vi "Joint Saturation Demo.vi"(10 "Joint Bounds [Deg/mm]":dbl[][](array[numeric])=[[-10.0, 35.0, 0.0, 0.0], [-35.0, -35.0, 0.0, 0.0], [0.5, 10.0, 0.0, 0.0], [-40.0, 40.0, 0.0, 0.0]], 11 "Ref Array [Deg/mm]":dbl[](array[numeric])=[0.0, 0.0, 0.0, 0.0]) -> (2 "Out of Bound?":bool, 3 "Sat Ref Array [Deg/mm]":dbl[](array[numeric]))   [LabVIEW 2016]
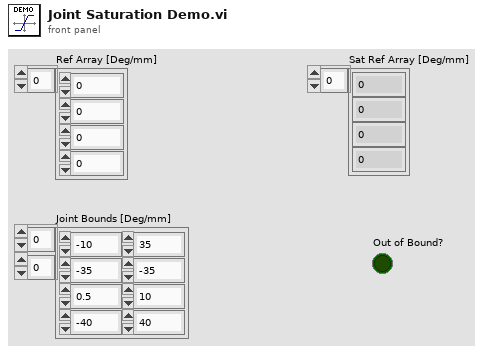
[diagram p1: front panel]
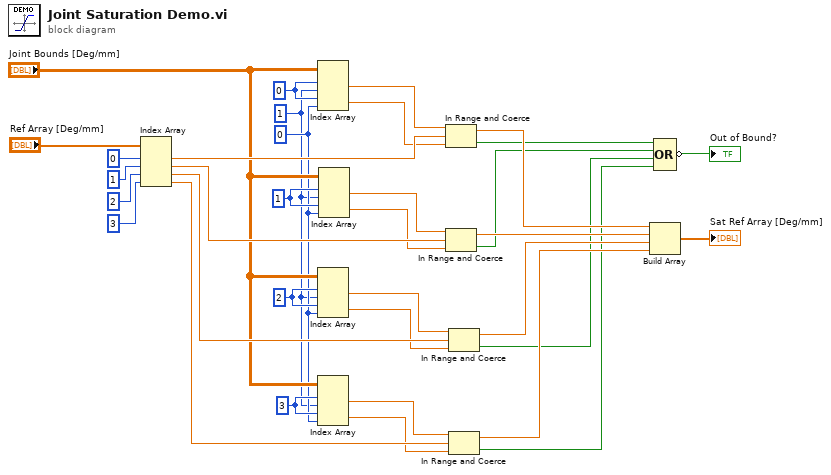
[diagram p0: block diagram]
diagram:
  w10 = 3 ("index (row)")
  w14 = 2
  w21 = 1 ("index (row)")
  w8 = 1 ("disabled index (col)")
  w9 = 0 ("index")
  w25 = 0 ("index")
  n1 = Index Array(array="Ref Array [Deg/mm]", index #1=0 ("index"), index #2=1 ("index"), index #3=2 ("index"), index #4=3 ("index")) -> (element #1=w29:dbl, element #2=w28:dbl, element #3=w27:dbl, element #4=w26:dbl)
  n2 = Index Array(array="Joint Bounds [Deg/mm]", index (row) #1=w25, index (col) #1=w8, index (row) #2=w25, index (col) #2=w9) -> (element #1=w24:dbl, element #2=w23:dbl)
  n3 = Index Array(array="Joint Bounds [Deg/mm]", index (row) #1=w14, index (col) #1=w8, index (row) #2=w14, index (col) #2=w9) -> (element #1=w13:dbl, element #2=w12:dbl)
  n4 = Index Array(array="Joint Bounds [Deg/mm]", index (row) #1=w10, index (col) #1=w8, index (row) #2=w10, index (col) #2=w9) -> (element #1=w7:dbl, element #2=w6:dbl)
  n5 = Index Array(array="Joint Bounds [Deg/mm]", index (row) #1=w21, index (col) #1=w8, index (row) #2=w21, index (col) #2=w9) -> (element #1=w20:dbl, element #2=w19:dbl)
  n6 = In Range and Coerce(upper limit=w24, x=w29, lower limit=w23) -> (coerced(x)=w22:dbl, In Range?=w4:bool)
  n7 = In Range and Coerce(upper limit=w20, x=w28, lower limit=w19) -> (coerced(x)=w17:dbl, In Range?=w3:bool)
  n8 = In Range and Coerce(upper limit=w13, x=w27, lower limit=w12) -> (coerced(x)=w16:dbl, In Range?=w2:bool)
  n9 = In Range and Coerce(upper limit=w7, x=w26, lower limit=w6) -> (coerced(x)=w15:dbl, In Range?=w1:bool)
  n10 = Build Array(w22, w17, w16, w15) -> (→"Sat Ref Array [Deg/mm]":dbl[])
  n11 = Compound Arithmetic op=OR(w4, w3, w2, w1) -> (invert →"Out of Bound?":bool)
